vi "Inst_Pistofono.vi"(8 "error in":errorcluster, 10 "All Message Queues in":T1, 11 "AjustesPrevios in":refnum<class "AjustesPrevios.lvclass">) -> (0 "error out":errorcluster)   [LabVIEW 2019, in "AjustesPrevios.lvclass"]
uses:
  AjustesPrevios.lvclass
  QMH/Message Queue/All Message Queues.ctl
  QMH/Message Queue/Message Cluster.ctl
  AjustesPrevios.lvclass/AjustesPrevios.ctl
  Instrumento/Pistofono/Pistofono.lvclass
  Controles/ClusterLecturaPistofono.ctl
  <vilib>/numeric/Random Number (Range) DBL.vi
  <vilib>/Utility/error.llb/Error Cluster From Error Code.vi
  QMH/Message Queue/Enqueue Message (Single).vi
  <vilib>/ErrorRing/Error Ring.xnode
  QMH/Message Queue/Message Queue.lvlib
panel:
  out "All States":string[](array[string])
  out "Actual State":string
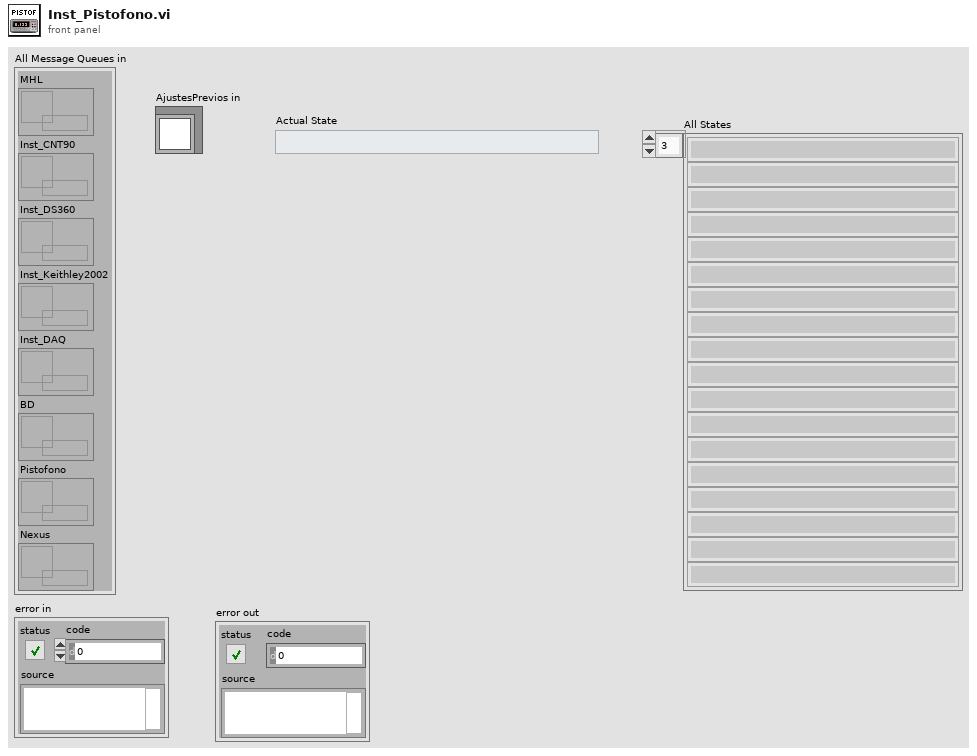
[diagram p1: front panel]
types:
  T1 = typedef "Message Queue.lvlib/All Message Queues.ctl" = cluster{"MHL":refnum<queue>, "Inst_CNT90":refnum<queue>, "Inst_DS360":refnum<queue>, "Inst_Keithley2002":refnum<queue>, "Inst_DAQ":refnum<queue>, "BD":refnum<queue>, "Pistofono":refnum<queue>, "Nexus":refnum<queue>}
  T2 = typedef "AjustesPrevios.lvclass/ClusterLecturaPistofono.ctl" = cluster{"temperatura":dbl, "presion":dbl, "nivel_emitido":dbl}
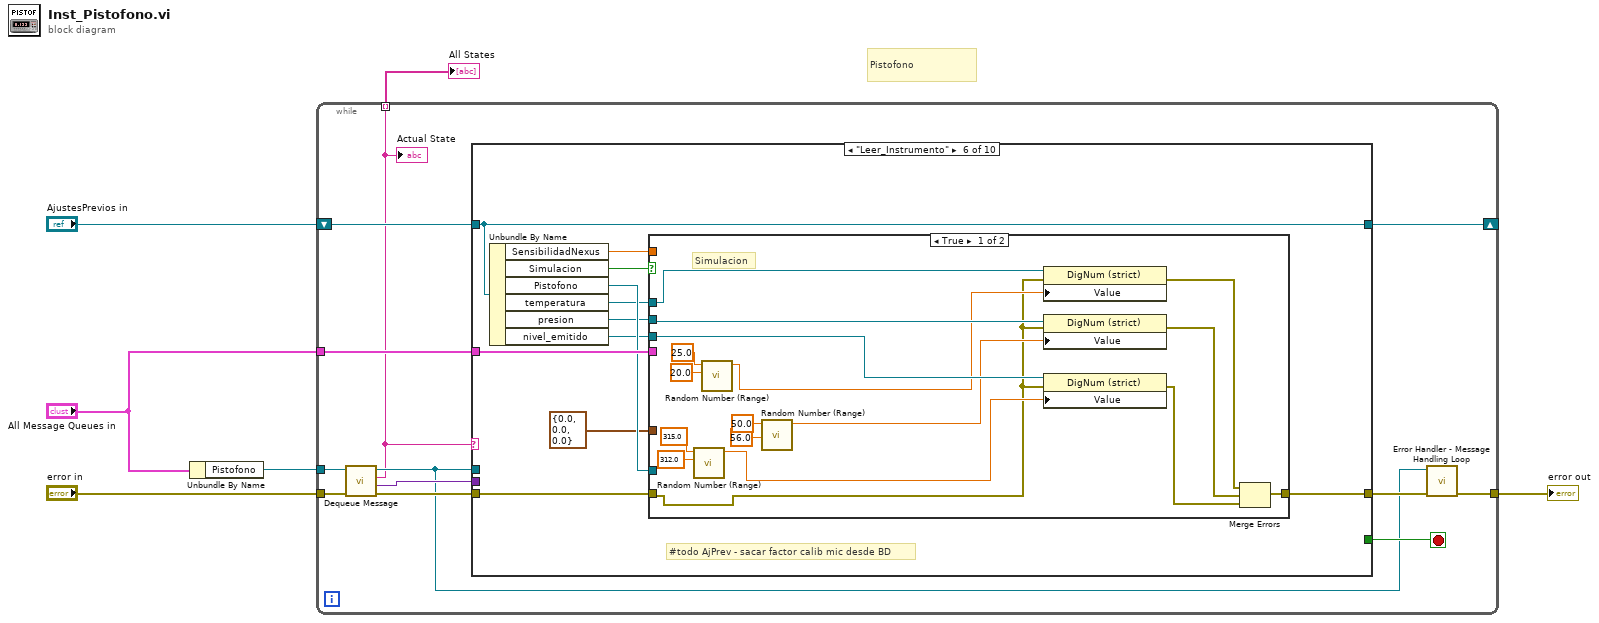
[diagram p0: block diagram]
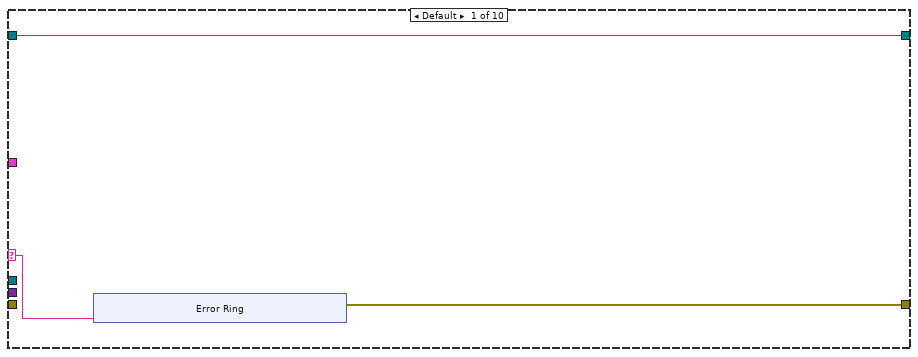
[diagram p2: hidden frame]
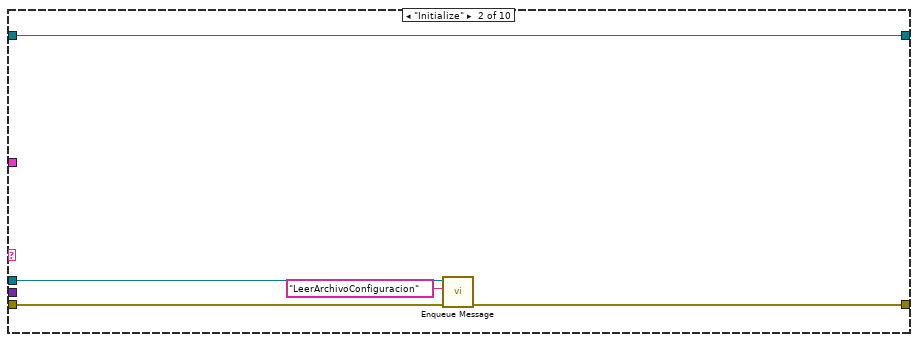
[diagram p3: hidden frame]
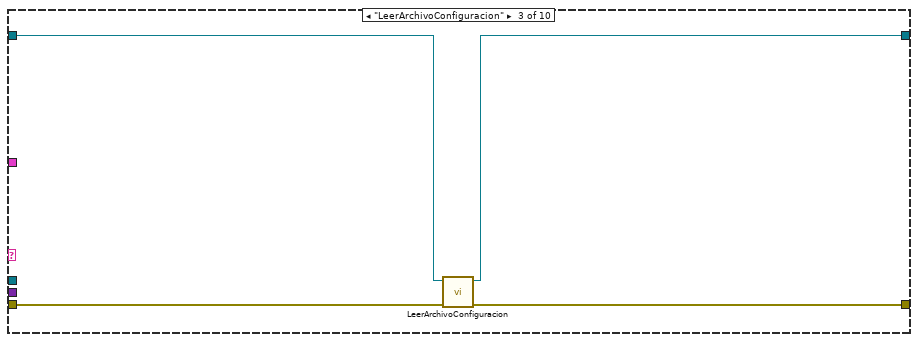
[diagram p4: hidden frame]
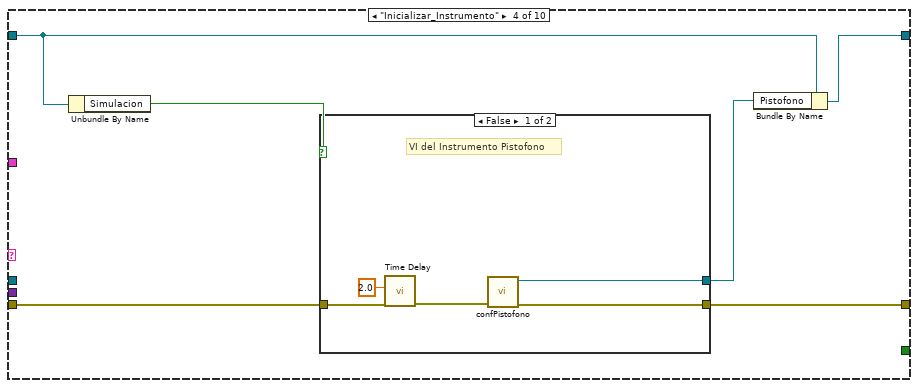
[diagram p5: hidden frame]
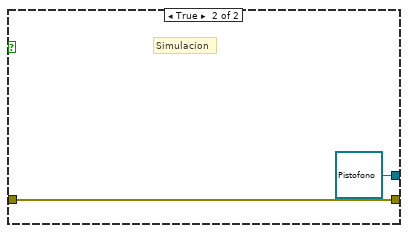
[diagram p6: hidden frame]
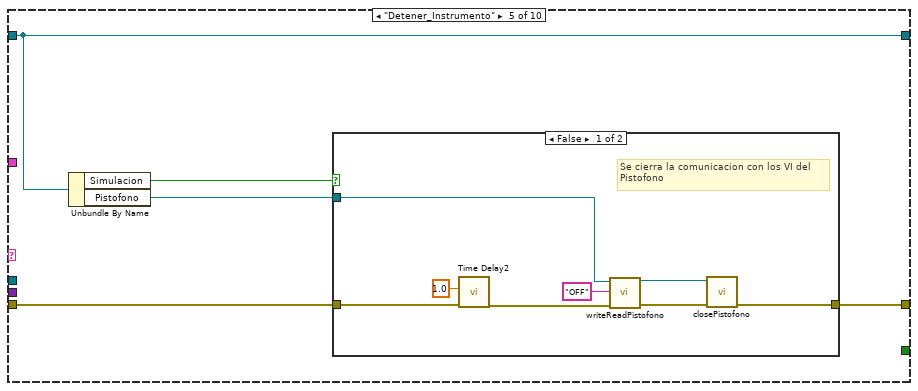
[diagram p7: hidden frame]
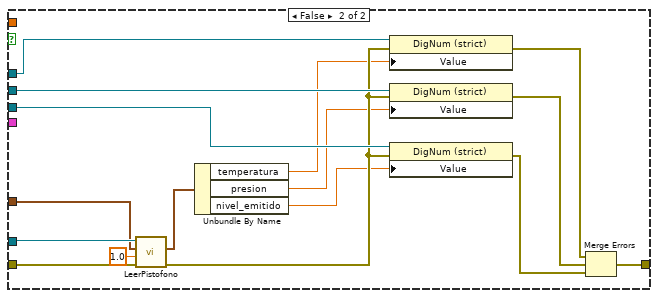
[diagram p9: hidden frame]
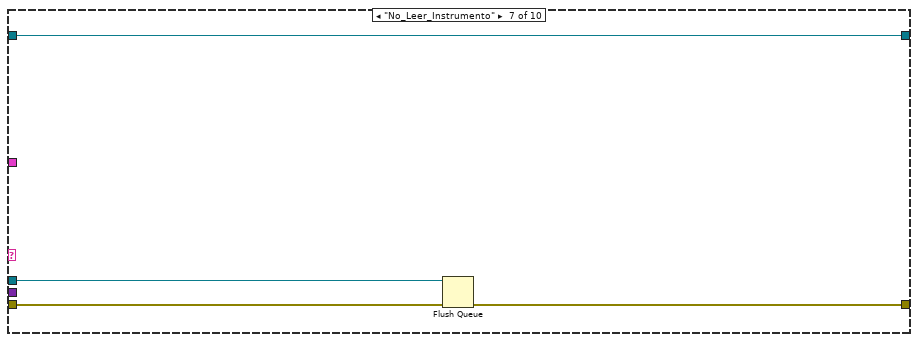
[diagram p10: hidden frame]
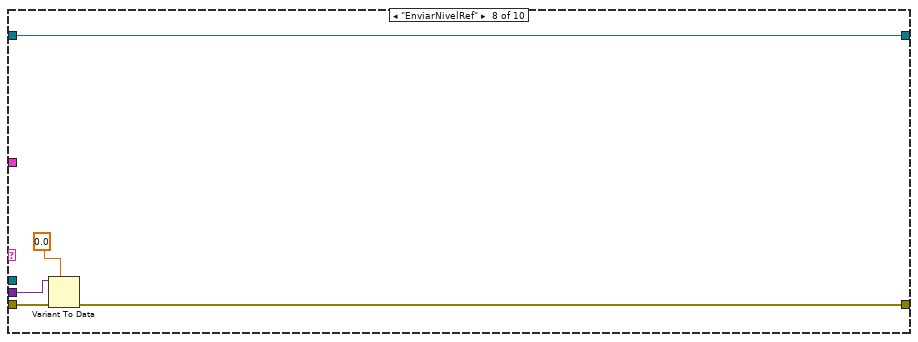
[diagram p11: hidden frame]
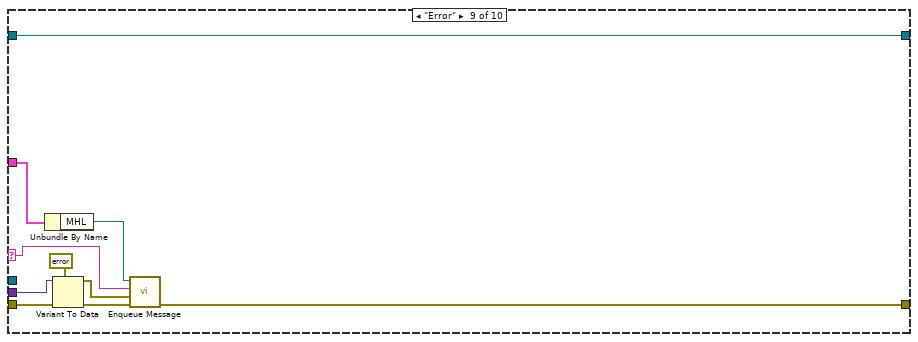
[diagram p12: hidden frame]
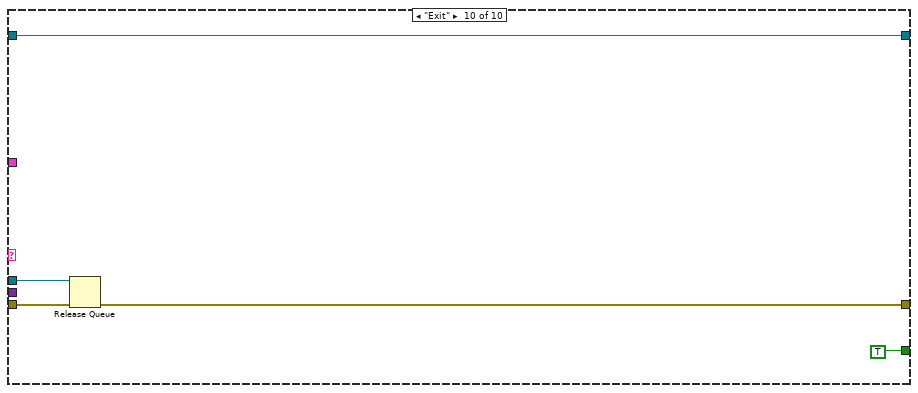
[diagram p13: hidden frame]
diagram:
  # "Pistofono"
  n1 = Unbundle By Name("All Message Queues in") -> ("Pistofono"=w4:refnum<queue>)
  n2 = while {
    tunnel: "error in" -> [w18]
    tunnel: w4 -> [w17]
    tunnel: "All Message Queues in" -> [w16]
    tunnel: [w9] -> w2
    shift-right: [w12] -> _
    shift-left: "AjustesPrevios in" -> [w15]
    tunnel: [w7] -> w1 mode=indexing
    stop <- w11 stop-if-true
    n3 = call "Dequeue Message.vi"("error in (no error)"=w18, "Message Queue"=w17) -> ("error out"=w13:errorcluster, "Message Data"=w14:variant, "Message"=w7:string, "dup Message Queue"=w8:refnum<queue>)  [unwired: 6 in]
    "Actual State" <- w7
    n4 = case shown="\"Leer_Instrumento\"" w7 {
      selector: w7 -> [w21 _ _ _ _ _ _ _ w120 _]
      tunnel: w16 -> [_ _ _ _ _ w73 _ _ w119 _]
      tunnel: w15 -> [w19 w33 w35 w40 w54 w75 w111 w113 w127 w129]
      tunnel: w8 -> [_ w30 _ _ _ _ w109 _ _ w131]
      tunnel: w14 -> [_ _ _ _ _ _ _ w114 w124 _]
      tunnel: w13 -> [_ w32 w37 w41 w52 w72 w112 w116 w125 w132]
      tunnel: [w20 w31 w36 w43 w55 w71 w110 w117 w122 w128] -> w10
      tunnel: [w19 w33 w34 w39 w54 w75 w111 w113 w127 w129] -> w12
      tunnel: [_ _ _ _ _ _ _ _ _ TRUE] -> w11
      frame Default {
        n5 = xnode "Error Ring"("parameter 0"=w21) -> ("error out"=w20:errorcluster)
      }
      frame "Initialize" {
        n6 = call-poly "Enqueue Message.vi"("error in (no error)"=w32, "Message"="LeerArchivoConfiguracion", "Message Queue"=w30) -> ("error out"=w31:errorcluster)  [unwired: 7 in, 1 out]
      }
      frame "LeerArchivoConfiguracion" {
        n7 = call "LeerArchivoConfiguracion.vi"("error in"=w37, "AjustesPrevios in"=w35) -> ("error out"=w36:errorcluster, "AjustesPrevios out"=w34:refnum<class "AjustesPrevios.lvclass">)  [unwired: 8 in]
      }
      frame "Inicializar_Instrumento" {
        n8 = Unbundle By Name(w40) -> ("Simulacion"=w42:bool)
        n9 = case shown="False" w42 {
          tunnel: [w48 w50] -> w43
          tunnel: w41 -> [w46 w50]
          tunnel: [w47 refnum<class "Pistofono.lvclass"> refnum ("Pistofono out")] -> w38
          frame False {
            # "VI del Instrumento Pistofono"
            n10 = call "Time Delay"("error in (no error)"=w46, "Delay Time (s)"=2.0) -> ("error out"=w45:errorcluster)  [unwired: 9 in]
            n11 = call "confPistofono.vi"("error in (no error)"=w45) -> ("error out"=w48:errorcluster, "Pistofono out"=w47:refnum<class "Pistofono.lvclass">)  [unwired: 8 in, 1 out]
          }
          frame True {
            # "Simulacion"
          }
        }
        n12 = Bundle By Name(cluster=w40, "Pistofono"=w38) -> (w39:refnum<class "AjustesPrevios.lvclass">)
      }
      frame "Detener_Instrumento" {
        n13 = Unbundle By Name(w54) -> ("Simulacion"=w53:bool, "Pistofono"=w51:refnum<class "Pistofono.lvclass">)
        n14 = case shown="False" w53 {
          tunnel: [w63 w64] -> w55
          tunnel: w52 -> [w59 w64]
          tunnel: w51 -> [w58 _]
          frame False {
            # "Se cierra la comunicacion con los VI del\nPistofono"
            n15 = call "Time Delay2"("error in (no error)"=w59, "Delay Time (s)"=1.0) -> ("error out"=w57:errorcluster)  [unwired: 9 in]
            n16 = call "writeReadPistofono.vi"("error in (no error)"=w57, "Command"="OFF", "Pistofono in"=w58) -> ("error out"=w60:errorcluster, "Pistofono out"=w61:refnum<class "Pistofono.lvclass">)  [unwired: 6 in, 1 out]
            n17 = call "closePistofono.vi"("error in (no error)"=w60, "Pistofono in"=w61) -> ("error out"=w63:errorcluster)  [unwired: 8 in, 1 out]
          }
          frame True {
            # "Simulacion"
          }
        }
      }
      frame "Leer_Instrumento" {
        # "#todo AjPrev - sacar factor calib mic desde BD"
        n18 = Unbundle By Name(w75) -> ("SensibilidadNexus"=w70:dbl, "Simulacion"=w74:bool, "Pistofono"=w69:refnum<class "Pistofono.lvclass">, "temperatura"=w67:refnum<vi>, "presion"=w66:refnum<vi>, "nivel_emitido"=w65:refnum<vi>)
        n19 = case shown="True" w74 {
          tunnel: w73 -> [_ _]
          tunnel: [w89 w96] -> w71
          tunnel: w72 -> [w76 w108]
          tunnel: w70 -> [_ _]
          tunnel: w69 -> [_ w107]
          tunnel: T2 {"temperatura"=0.0, "presion"=0.0, "nivel_emitido"=0.0} ("clusterPistofono") -> [_ w106]
          tunnel: w67 -> [w88 w103]
          tunnel: w66 -> [w87 w102]
          tunnel: w65 -> [w86 w101]
          frame True {
            # "Simulacion"
            n20 = call-poly <vilib>:"Random Number (Range).vi"("lower bound (0)"=312.0, "upper bound (100)"=315.0) -> ("number"=w77:dbl)  [unwired: 9 in]
            n21 = call-poly <vilib>:"Random Number (Range).vi"("lower bound (0)"=20.0, "upper bound (100)"=25.0) -> ("number"=w79:dbl)  [unwired: 9 in]
            n22 = call-poly <vilib>:"Random Number (Range).vi"("lower bound (0)"=56.0, "upper bound (100)"=50.0) -> ("number"=w78:dbl)  [unwired: 9 in]
            n23 = property class="DigNum (strict)"(reference=w88, error in=w76, "Value"=w79) -> (error out=w92:errorcluster)  [unwired: 1 out]
            n24 = property class="DigNum (strict)"(reference=w87, error in=w76, "Value"=w78) -> (error out=w90:errorcluster)  [unwired: 1 out]
            n25 = property class="DigNum (strict)"(reference=w86, error in=w76, "Value"=w77) -> (error out=w91:errorcluster)  [unwired: 1 out]
            n26 = Merge Errors(w92, w90, w91) -> (w89:errorcluster)
          }
          frame False {
            n27 = call "LeerPistofono.vi"("error in (no error)"=w108, "FactorCalibPistofono"=1.0, "clusterPistofono"=w106, "Pistofono in"=w107) -> ("error out"=w100:errorcluster, "clusterPistofono out"=w104:T2)  [unwired: 5 in, 1 out]
            n28 = Unbundle By Name(w104) -> ("temperatura"=w99:dbl, "presion"=w98:dbl, "nivel_emitido"=w97:dbl)
            n29 = property class="DigNum (strict)"(reference=w103, error in=w100, "Value"=w99) -> (error out=w95:errorcluster)  [unwired: 1 out]
            n30 = property class="DigNum (strict)"(reference=w102, error in=w100, "Value"=w98) -> (error out=w93:errorcluster)  [unwired: 1 out]
            n31 = property class="DigNum (strict)"(reference=w101, error in=w100, "Value"=w97) -> (error out=w94:errorcluster)  [unwired: 1 out]
            n32 = Merge Errors(w95, w93, w94) -> (w96:errorcluster)
          }
        }
      }
      frame "No_Leer_Instrumento" {
        n33 = Flush Queue(queue=w109, error in (no error)=w112) -> (error out=w110:errorcluster)  [unwired: 2 out]
      }
      frame "EnviarNivelRef" {
        n34 = Variant To Data(error in=w116, type=0.0, Variant=w114) -> (error out=w117:errorcluster)  [unwired: 1 out]
      }
      frame "Error" {
        n35 = Unbundle By Name(w119) -> ("MHL"=w118:refnum<queue>)
        n36 = Variant To Data(error in=w125, type=errorcluster {"status"=FALSE, "code"=0, "source"=""} ("error constant"), Variant=w124) -> (data=w121:errorcluster, error out=w123:errorcluster)
        n37 = call-poly "Enqueue Message.vi"("error in (no error)"=w123, "Message Data"=w121, "Message"=w120, "Message Queue"=w118) -> ("error out"=w122:errorcluster)  [unwired: 6 in, 1 out]
      }
      frame "Exit" {
        n38 = Release Queue(queue=w131, error in (no error)=w132) -> (error out=w128:errorcluster)  [unwired: 1 in, 2 out]
      }
    }
    n39 = call "Error Handler - Message Handling Loop.vi"("error in (no error)"=w10, "Message Queue"=w8) -> ("dup error in"=w9:errorcluster)  [unwired: 8 in, 1 out]
  }
  "error out" <- w2
  "All States" <- w1
